vi "读取电子表格文件.vi"() -> ()   [LabVIEW 2010]
uses:
  <vilib>/Utility/file.llb/Read From Spreadsheet File (DBL).vi
panel:
  out "读取数据显示":dbl[][](graph)
  in  "偏移量":i32
  in  "读取数据行数":i32=-1
  in  "文件路径及名称":path
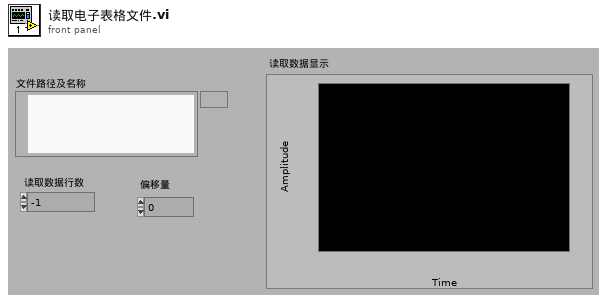
[diagram p1: front panel]
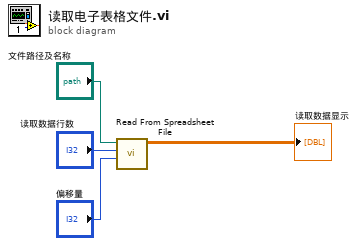
[diagram p0: block diagram]
diagram:
  n1 = call-poly <vilib>:"Read From Spreadsheet File.vi"("start of read offset (chars.:0)"="偏移量", "number of rows (all:-1)"="读取数据行数", "file path (dialog if empty)"="文件路径及名称") -> ("all rows"=→"读取数据显示":dbl[][])  [unwired: 4 in, 4 out]
